vi "Extract Sentences.vi"(8 "error in (no error)":errorcluster, 9 "filter for sentence type":string, 10 "sensor data":string, 11 "previous partial sentence":string) -> (0 "error out":errorcluster, 2 "complete sentences":string[](array[string]), 3 "remaining partial sentence":string, 4 "invalid sentences":string[](array[string]), 5 "discarded data before first sentence":string)   [LabVIEW 2024]
uses:
  <vilib>/regexp/Match Regular Expression.xnode
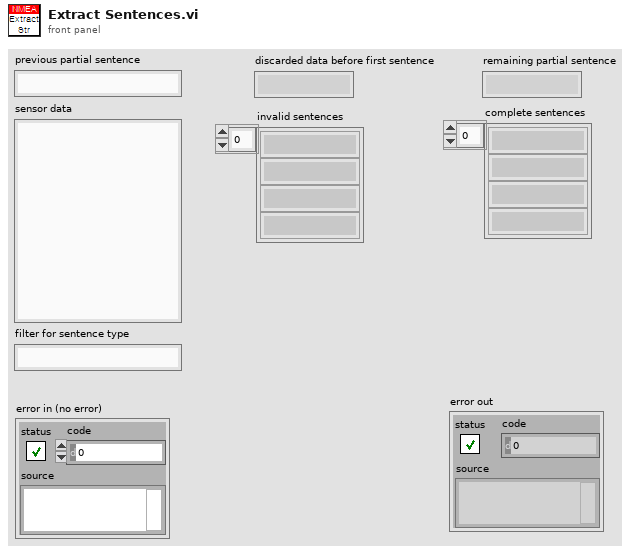
[diagram p1: front panel]
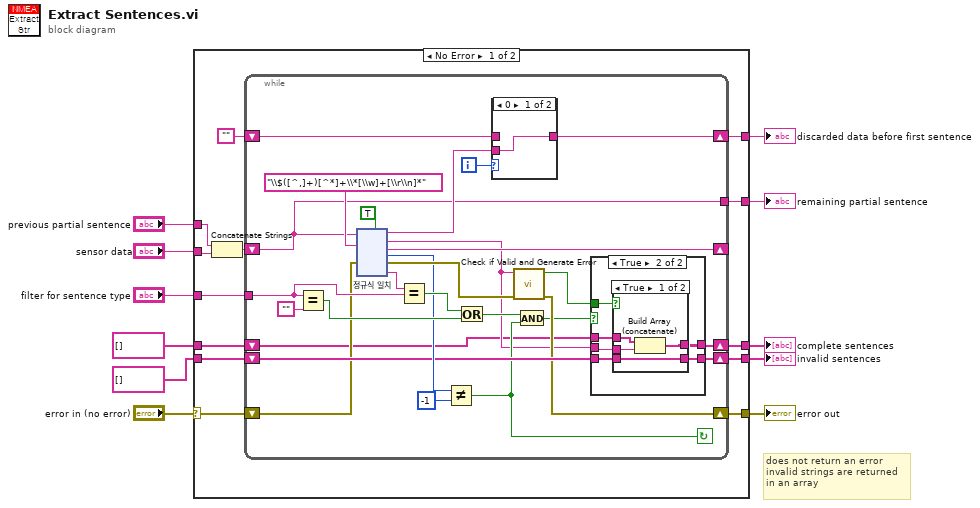
[diagram p0: block diagram]
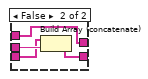
[diagram p3: hidden frame]
diagram:
  # "does not return an error\ninvalid strings are returned\nin an array"
  n1 = case shown="No Error" "error in (no error)" {
    selector: "error in (no error)" -> [w18 w191]
    tunnel: [w17 w191] -> w10
    tunnel: "previous partial sentence" -> [w14 _]
    tunnel: [w21 _] -> w8
    tunnel: "filter for sentence type" -> [w24 _]
    tunnel: "sensor data" -> [w15 _]
    tunnel: string[] [] -> [w23 w190]
    tunnel: [w22 w190] -> w4
    tunnel: string[] [] -> [w20 w189]
    tunnel: [w19 w189] -> w2
    tunnel: [w12 _] -> w1
    frame No Error {
      n2 = Concatenate Strings(w14, w15) -> (w16:string)
      n3 = while {
        tunnel: w24 -> [w44]
        shift-right: [w41] -> w22
        shift-left: w23 -> [w25]
        shift-right: [w48] -> _
        shift-left: w16 -> [w30]
        tunnel: [w30] -> w21
        shift-right: [w35] -> w19
        shift-left: w20 -> [w36]
        shift-right: [w33] -> w17
        shift-left: w18 -> [w34]
        shift-right: [w27] -> w12
        shift-left: "" -> [w28]
        i -> [w51]
        stop <- w31 continue-if-true
        n4 = Equal?(x=w44, y="") -> (x = y?=w42:bool)
        n5 = xnode "정규식 일치"("입력 문자열"=w30, "정규식"="\\$([^,]+)[^*]+\\*[\\w]+[\\r\\n]*" ("regular expression"), "에러 입력"=w34, "여러 라인? (거짓)"=TRUE) -> ("일치 구문 앞"=w49:string, "전체 일치 구문"=w26:string, "일치 구문 뒤"=w48:string, "일치 구문 뒤의 오프셋"=w40:i32, "에러 출력"=w47:errorcluster, "부분 일치 1"=w45:string)  [unwired: 1 in, 1 out]
        n6 = Equal?(x=w45, y=w44) -> (x = y?=w43:bool)
        n7 = Not Equal?(x=w40, y=-1) -> (x != y?=w31:bool)
        n8 = Or(x=w43, y=w42) -> (x .or. y?=w38:bool)
        n9 = case shown="0" w51 {
          tunnel: w49 -> [w68 _]
          tunnel: w28 -> [_ w69]
          tunnel: [w68 w69] -> w27
          frame 0 {
          }
          frame 1, Default {
          }
        }
        n10 = call "Check if Valid and Generate Error.vi"("error in (no error)"=w47, "sentence"=w26) -> ("error out"=w33:errorcluster, "valid sentence"=w37:bool)  [unwired: 8 in]
        n11 = And(x=w38, y=w31) -> (x .and. y?=w32:bool)
        n12 = case shown="True" w32 {
          tunnel: w25 -> [w53 w59]
          tunnel: w26 -> [_ w58]
          tunnel: [w53 w57] -> w41
          tunnel: w37 -> [_ w56]
          tunnel: w36 -> [w52 w55]
          tunnel: [w52 w54] -> w35
          frame False {
          }
          frame True {
            n13 = case shown="True" w56 {
              tunnel: w59 -> [w63 w64]
              tunnel: w58 -> [w62 w67]
              tunnel: [w61 w64] -> w57
              tunnel: w55 -> [w60 w66]
              tunnel: [w60 w65] -> w54
              frame True {
                n14 = Build Array (concatenate)(w63, w62) -> (w61:string[])
              }
              frame False {
                n15 = Build Array (concatenate)(w66, w67) -> (w65:string[])
              }
            }
          }
        }
      }
    }
    frame Error {
    }
  }
  "complete sentences" <- w4
  "remaining partial sentence" <- w8
  "error out" <- w10
  "invalid sentences" <- w2
  "discarded data before first sentence" <- w1
